vi "CALC_MARK_FUNC_EXEC.vi"(0 "VISA IN":refnum<visa-resource-name>, 1 "Marker number":i32, 2 "Function":string(combo)="MAX", 5 "error in":errorcluster, 7 "Channel":i32) -> (14 "VISA Out":refnum<visa-resource-name>, 19 "error out":errorcluster)   [LabVIEW 2018, in "PNA-X.lvlib"]
doc: "CALCulate<cnum>:MARKer<mkr>:FUNCtion:EXECute [<func>] \n(Write-only) Immediately executes (performs) the specified search function. If no function is \nspecified, executes the selected function. Select the function with CALC:MARK:FUNCtion:SEL. \nSee Critical Note \nParameters \n<cnum> Channel number of the measurement. There must be a selected measurement \non that channel. If unspecified, <cnum> is set to 1. \n<mkr> Any marker number from 1 to 10; if unspecified, value is set to 1. \n<func> Optional argument. The function that is to be performed. Choose from: \nMAXimum - finds the highest value \nMINimum - finds the lowest value \nRPEak - finds the next valid peak to the right \nLPEak - finds the next valid peak to the left \nNPEak - finds the next highest value among the valid peaks \nTARGet - finds the target value to the right, wraps around to the left \nLTARget - finds the next target value to the left of the marker \nRTARget - finds the next target value to the right of the marker \n1536\n\nExamples CALC:MARK:FUNC:EXEC \ncalculate2:marker2:function:execute maximum \nQuery Syntax Not applicable \nDefault Not applicable"
uses:
  PNA-X.lvlib
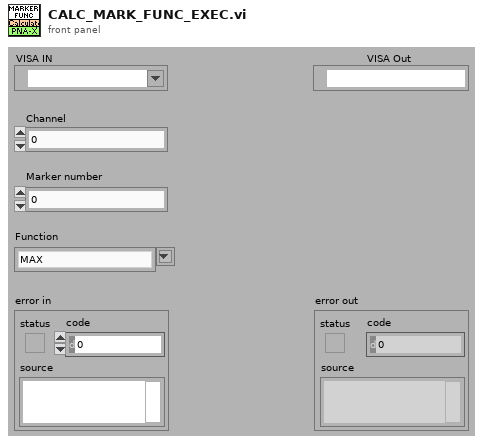
[diagram p1: front panel]
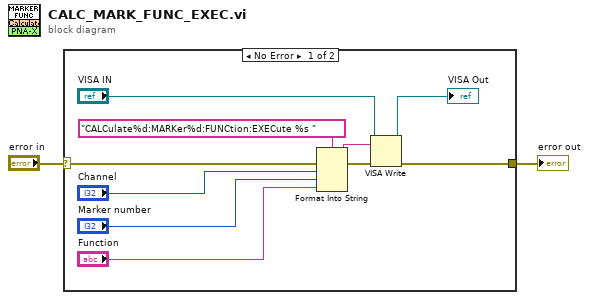
[diagram p0: block diagram]
diagram:
  n1 = case shown="No Error" "error in" {
    selector: "error in" -> [w12 w13]
    tunnel: [w7 w13] -> w1
    frame No Error {
      n2 = Format Into String(format string="CALCulate%d:MARKer%d:FUNCtion:EXECute %s " ("Cmdline"), error in=w12, "Channel", "Marker number", "Function") -> (resulting string=w10:string, error out=w11:errorcluster)  [unwired: 1 in]
      n3 = VISA Write(VISA resource name="VISA IN", write buffer=w10, error in (no error)=w11) -> (VISA resource name out=→"VISA Out":refnum<visa-resource-name>, error out=w7:errorcluster)  [unwired: 1 out]
    }
    frame Error {
    }
  }
  "error out" <- w1
